vi "Init.vi"(8 "error in":errorcluster, 11 "TDMS Sink in":refnum<class "TDMS Sink.lvclass">) -> (0 "error out":errorcluster, 3 "TDMS Sink out":refnum<class "TDMS Sink.lvclass">)   [LabVIEW 2024, in "TDMS Sink.lvclass"]
uses:
  TDMS Sink.lvclass
  TDMS Sink.lvclass/TDMS Sink.ctl
  dd141f00-aa81-4722-bc7e-f0d40e96bd8b.vi
  dd141f00-aa81-4722-bc7e-f0d40e96bd8b.vi/a4169a97-72fc-4003-a778-603cf20cafa0.vi
  <vilib>/JDP Science/JSONtext/Find Item.vi
  <vilib>/JDP Science/JSONtext/Next JSON Value.vi
  <vilib>/JDP Science/JSONtext/String Subset.vi
  <vilib>/JDP Science/JSONtext/Parsing/Advance past next JSON Value (inlined COPY).vi
  <vilib>/JDP Science/JSONtext/Parsing/Advance past whitespace.vi
  <vilib>/JDP Science/JSONtext/Parsing/Advance past String.vi
  <vilib>/JDP Science/JSONtext/Parsing/Advance past Number.vi
  <vilib>/JDP Science/JSONtext/Parsing/Advance past Line Ending.vi
  <vilib>/JDP Science/JSONtext/Parsing/Parse Full Path or Item Name.vi
  <vilib>/JDP Science/JSONtext/Parsing/Advance past Array.vi
  <vilib>/JDP Science/JSONtext/Parsing/Advance past Object.vi
  <vilib>/JDP Science/JSONtext/support/Error Cluster From Code.vi
  <vilib>/JDP Science/JSONtext/Offset/Find Item Locations by Path.vi
  <vilib>/JDP Science/JSONtext/JSON text to Variant.vi
  <vilib>/Utility/error.llb/Error Cluster From Error Code.vi
  <vilib>/JDP Science/JSONtext/LVClass Serializer/JSONtext LVClass Serializer.lvclass
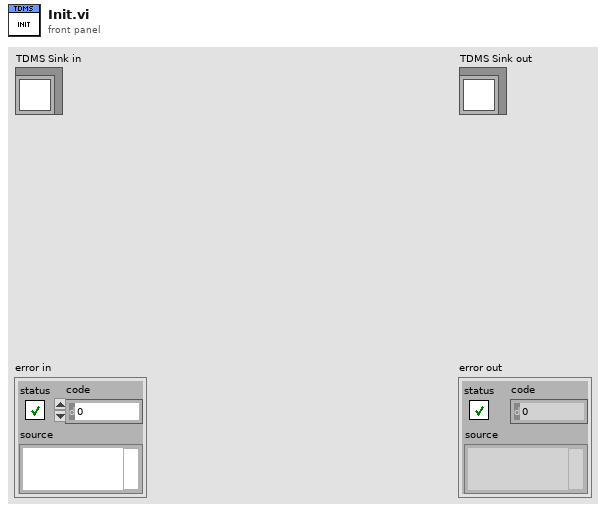
[diagram p1: front panel]
types:
  T1 = enum16{"open", "open or create", "create or replace", "create", "open (read-only)"}
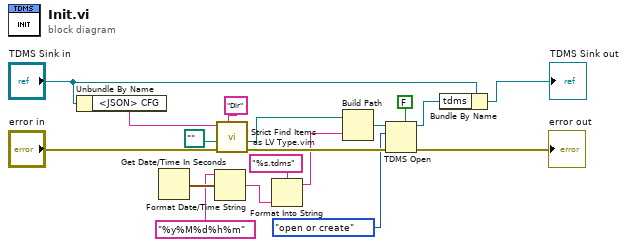
[diagram p0: block diagram]
diagram:
  n1 = Unbundle By Name("TDMS Sink in") -> ("<JSON> CFG"=w15:string)
  n2 = Get Date/Time In Seconds() -> (seconds since 1Jan1904=w9:timestamp)
  n3 = Format Date/Time String(time format string (%c)="%y%M%d%h%m", seconds (now)=w9) -> (date/time string=w3:string)  [unwired: 1 in]
  n4 = call "Strict Find Items as LV Type.vim"("$Path or Item Name"="Dir", "error in"="error in", "Data Type and Default Value"=path "", "<JSON>"=w15) -> ("error out"=w17:errorcluster, "Data out"=w10:path)  [unwired: 5 in, 1 out]
  n5 = Format Into String(format string="%s.tdms", w3) -> (resulting string=w1:string)  [unwired: 2 in, 1 out]
  n6 = Build Path(base path=w10, name or relative path=w1) -> (appended path=w11:path)
  n7 = TDMS Open(5:FALSE ("create index file? (T)"), 8:w17, 10:T1."open or create" ("operation (0:open)"), 11:w11) -> (0:→"error out":errorcluster, 3:w4:refnum<k34>)  [unwired: 3 in]
  n8 = Bundle By Name(cluster="TDMS Sink in", "tdms"=w4) -> (→"TDMS Sink out":refnum<class "TDMS Sink.lvclass">)
